vi "Create Wheel Angular Velocity Row.vi"(8 "error in (no error)":errorcluster, 10 "steering angle (rad)":dbl, 11 "caster wheel in":refnum<class "NI_Robotics_Caster Wheel.lvclass">) -> (0 "error out":errorcluster, 2 "wheel angular velocity row":dbl[](array[numeric]), 3 "caster wheel out":refnum<class "NI_Robotics_Caster Wheel.lvclass">)   [LabVIEW 2017, in "NI_Robotics_Caster Wheel.lvclass"]
uses:
  <vilib>/robotics/Steering/Caster Wheel/NI_Robotics_Caster Wheel.lvclass
  c:/Program Files (x86)/National Instruments/LabVIEW 2017/vi.lib/robotics/Steering/Wheel/NI_Robotics_Wheel.lvclass
  <vilib>/robotics/Steering/Wheel/NI_Robotics_Wheel.lvclass/NI_Robotics_Wheel.ctl
  <vilib>/robotics/Steering/Caster Wheel/NI_Robotics_Caster Wheel.lvclass/NI_Robotics_Caster Wheel.ctl
  <vilib>/robotics/Steering/Wheel/NI_Robotics_Wheel.lvclass
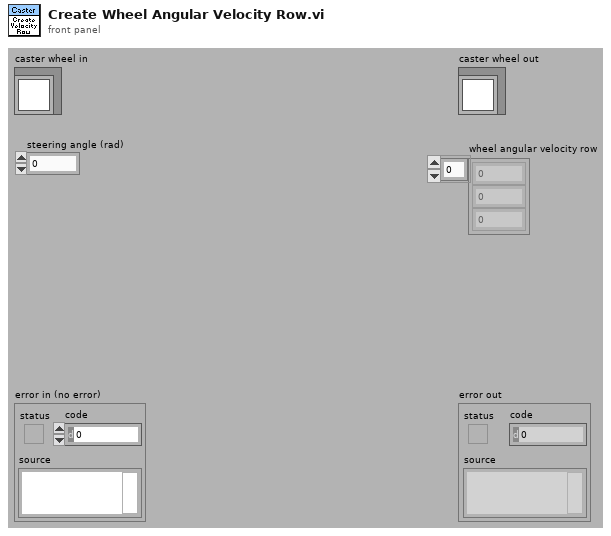
[diagram p1: front panel]
types:
  T1 = typedef "NI_Matrix.lvlib/RealMatrix.ctl" = dbl[][]
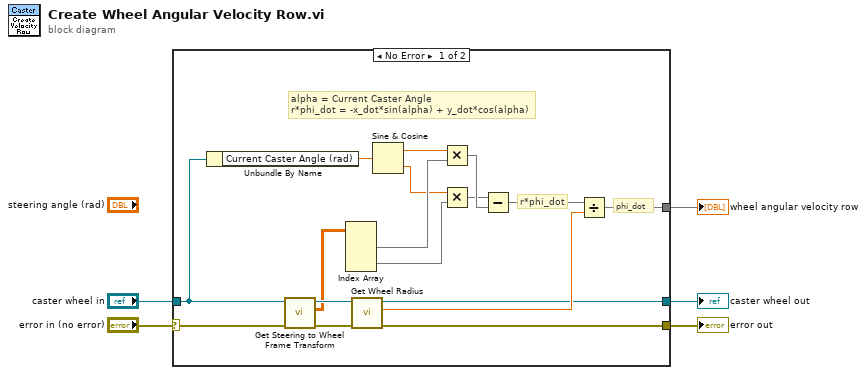
[diagram p0: block diagram]
diagram:
  n1 = case shown="No Error" "error in (no error)" {
    selector: "error in (no error)" -> [w11 w24]
    tunnel: [w16 w24] -> w4
    tunnel: "caster wheel in" -> [w13 w23]
    tunnel: [w15 w23] -> w2
    tunnel: [w14 _] -> w1
    frame No Error {
      # "phi_dot"
      # "r*phi_dot"
      # "alpha = Current Caster Angle\nr*phi_dot = -x_dot*sin(alpha) + y_dot*cos(alpha)"
      n2 = Unbundle By Name(w13) -> ("Current Caster Angle (rad)"=w8:dbl)
      n3 = call <vilib>:"Get Steering to Wheel Frame Transform.vi"("error in (no error)"=w11, "wheel in"=w13) -> ("error out"=w10:errorcluster, "steering to wheel frame transform"=w9:T1, "wheel out"=w12:refnum<class "NI_Robotics_Caster Wheel.lvclass">)  [unwired: 7 in]
      n4 = Index Array(array=w9) -> (element #1=w19:dbl[], element #2=w18:dbl[])  [unwired: 4 in]
      n5 = call <vilib>:"Get Wheel Radius.vi"("error in (no error)"=w10, "wheel in"=w12) -> ("error out"=w16:errorcluster, "wheel radius"=w17:dbl, "wheel out"=w15:refnum<class "NI_Robotics_Caster Wheel.lvclass">)  [unwired: 7 in]
      n6 = Sine & Cosine(0:w8) -> (1:w7:dbl, 2:w6:dbl)
      n7 = Multiply(x=w7, y=w19) -> (x*y=w21:dbl[])
      n8 = Multiply(x=w6, y=w18) -> (x*y=w20:dbl[])
      n9 = Subtract(x=w20, y=w21) -> (x-y=w22:dbl[])
      n10 = Divide(x=w22, y=w17) -> (x/y=w14:dbl[])
    }
    frame Error {
    }
  }
  "error out" <- w4
  "caster wheel out" <- w2
  "wheel angular velocity row" <- w1
